vi "mediaBalls_v2.vi"(7 "cameras array":dbl[](array[numeric]), 9 "Field Size":T2, 10 "grSim?":bool=TRUE, 11 "Array Ball Pose + CamID":T1(array[cluster])) -> (2 "No cameras?":bool, 3 "Ball out":cluster{"x":dbl, "y":dbl})   [LabVIEW 2018]
panel:
  out "Array":i32[](array[numeric])
  in  "Cam Intersection Widht":u32=6
  in  "Cam Intersection Lenght":u32=6
  in  "cluster":cluster{"x":dbl, "y":dbl}
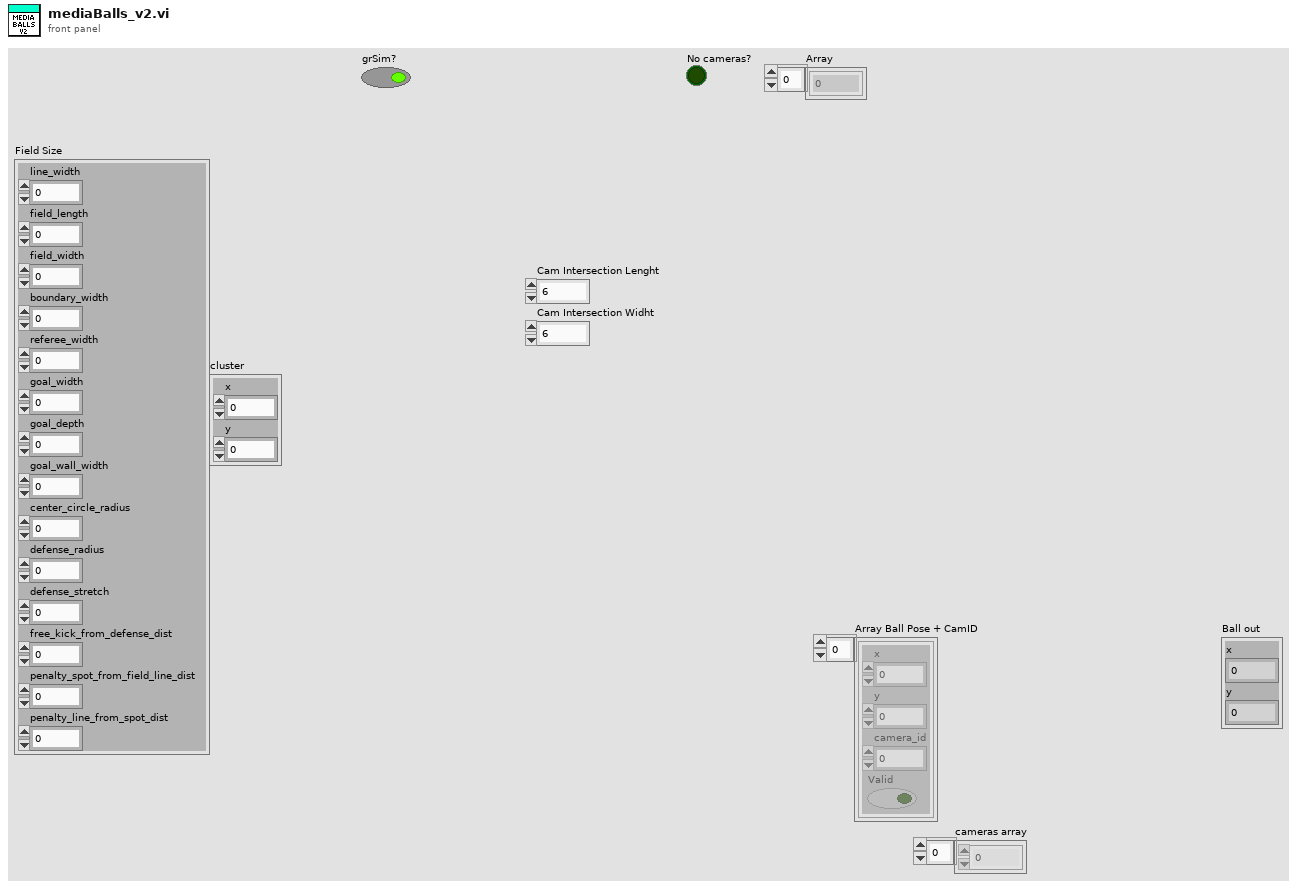
[diagram p1: front panel]
types:
  T1 = cluster{"x":sgl, "y":sgl, "camera_id":u32, "Valid":bool}[]
  T2 = cluster{"line_width":u32, "field_length":u32, "field_width":u32, "boundary_width":u32, "referee_width":u32, "goal_width":u32, "goal_depth":u32, "goal_wall_width":u32, "center_circle_radius":u32, "defense_radius":u32, "defense_stretch":u32, "free_kick_from_defense_dist":u32, "penalty_spot_from_field_line_dist":u32, "penalty_line_from_spot_dist":u32}
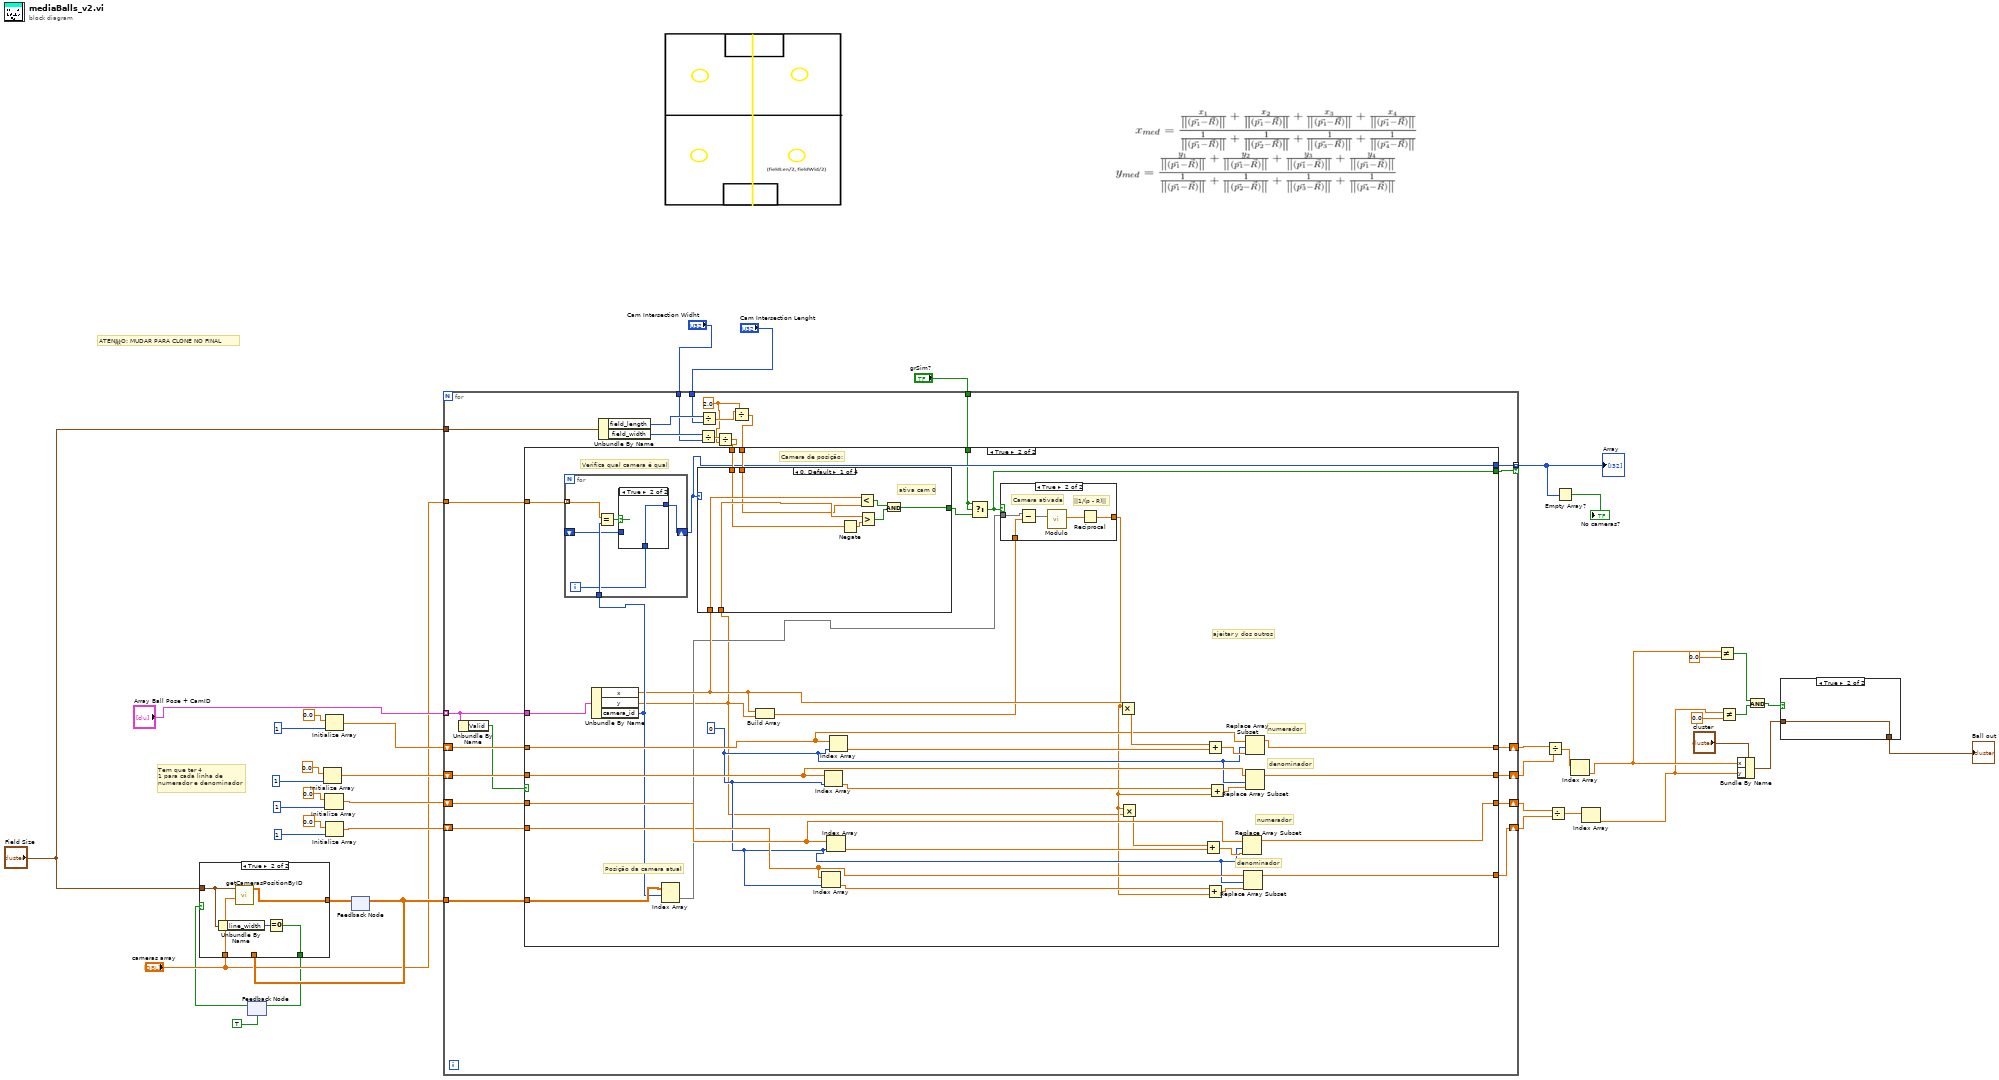
[diagram p0: block diagram]
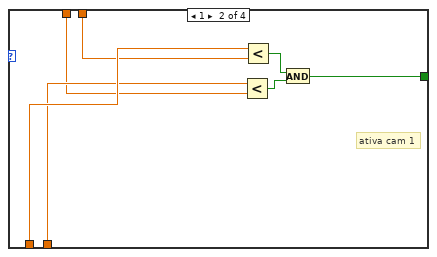
[diagram p5: hidden frame]
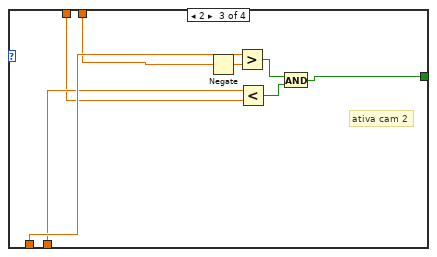
[diagram p6: hidden frame]
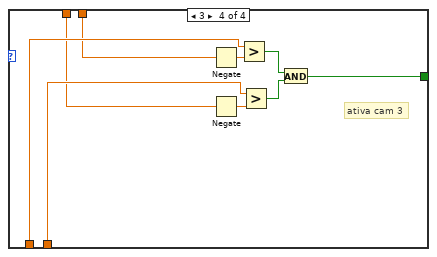
[diagram p7: hidden frame]
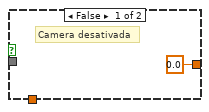
[diagram p9: hidden frame]
diagram:
  # "Tem que ter 4\n1 para cada linha de\nnumerador e denominador"
  # "ATEN敲O: MUDAR PARA CLONE NO FINAL"
  n1 = feedback #1(TRUE) -> (w2:bool)
  n2 = Initialize Array(0.0 ("element"), 1 ("dimension size")) -> (w32:dbl[])
  n3 = Initialize Array(0.0 ("element"), 1 ("dimension size")) -> (w31:dbl[])
  n4 = Initialize Array(0.0 ("element"), 1 ("dimension size")) -> (w33:dbl[])
  n5 = Initialize Array(0.0 ("element"), 1 ("dimension size")) -> (w30:dbl[])
  n6 = feedback #2() -> (w11:dbl[][])  [unwired: 1 in]
  n7 = case shown="True" w2 {
    selector: w2 -> [w42 _]
    tunnel: "Field Size" -> [_ w46]
    tunnel: [w43 w48] -> w12
    tunnel: w11 -> [w43 _]
    tunnel: "cameras array" -> [_ w47]
    tunnel: [w42 w44] -> w1
    frame False {
    }
    frame True {
      n8 = Unbundle By Name(w46) -> ("line_width"=w45:u32)
      n9 = call "getCamerasPositionByID.vi"("cameras id"=w47, "Field Size 2"=w46) -> ("Cameras Positions"=w48:dbl[][])  [unwired: 9 in]
      n10 = Equal To 0?(x=w45) -> (x = 0?=w44:bool)
    }
  }
  n11 = feedback-in #1(w1) -> ()
  n12 = feedback-in #2(w12) -> ()
  n13 = for {
    tunnel: "Array Ball Pose + CamID" -> [w50] mode=indexing
    tunnel: w11 -> [w73]
    shift-right: [w72] -> w29
    shift-left: w33 -> [w66]
    shift-right: [w71] -> w28
    shift-left: w32 -> [w65]
    shift-right: [w70] -> w27
    shift-left: w31 -> [w68]
    shift-right: [w69] -> w26
    shift-left: w30 -> [w67]
    tunnel: "cameras array" -> [w64]
    tunnel: "Cam Intersection Widht" -> [w61]
    tunnel: "Cam Intersection Lenght" -> [w60]
    tunnel: "Field Size" -> [w59]
    tunnel: "grSim?" -> [w58]
    tunnel: [w57] -> w7 mode=indexing if=w56
    w51 = 2.0
    n14 = Unbundle By Name(w50) -> ("Valid"=w49:bool)
    n15 = Unbundle By Name(w59) -> ("field_length"=w63:u32, "field_width"=w62:u32)
    n16 = Divide(x=w62, y=w61) -> (x/y=w53:dbl)
    n17 = Divide(x=w63, y=w60) -> (x/y=w55:dbl)
    n18 = Divide(x=w53, y=w51) -> (x/y=w52:dbl)
    n19 = Divide(x=w55, y=w51) -> (x/y=w54:dbl)
    n20 = case shown="True" w49 {
      tunnel: w73 -> [_ w111]
      tunnel: [w77 w101] -> w72
      tunnel: [w76 w100] -> w71
      tunnel: [w75 w99] -> w70
      tunnel: [w74 w98] -> w69
      tunnel: w68 -> [w75 w97]
      tunnel: w67 -> [w74 w96]
      tunnel: w66 -> [w77 w95]
      tunnel: w65 -> [w76 w94]
      tunnel: w50 -> [_ w91]
      tunnel: w64 -> [_ w89]
      tunnel: w52 -> [_ w88]
      tunnel: w54 -> [_ w87]
      tunnel: w58 -> [_ w80]
      tunnel: [_ w81] -> w57
      tunnel: [_ w78] -> w56
      frame False {
      }
      frame True {
        w93 = 0 ("index")
        # "Verifica qual camera é qual"
        # "Camera de posição:"
        # "ajeitar y dos outros"
        # "denominador"
        # "numerador"
        # "denominador"
        # "numerador"
        # "Posição da camera atual"
        n21 = Unbundle By Name(w91) -> ("x"=w86:sgl, "y"=w82:sgl, "camera_id"=w90:u32)
        n22 = for {
          tunnel: w90 -> [w149]
          shift-right: [w146] -> w81
          shift-left: _ -> [w145]
          tunnel: w89 -> [w144] mode=indexing
          i -> [w147]
          n23 = Equal?(x=w144, y=w149) -> (x = y?=w148:bool)
          n24 = case shown="True" w148 {
            tunnel: w147 -> [_ w151]
            tunnel: [w150 w151] -> w146
            tunnel: w145 -> [w150 _]
            frame False {
            }
            frame True {
            }
          }
        }
        n25 = Index Array(array=w111, index (row)=w90) -> (element=w85:dbl[])  [unwired: 1 in]
        n26 = case shown="0, Default" w81 {
          tunnel: w86 -> [w116 w124 w131 w139]
          tunnel: w82 -> [w115 w123 w130 w138]
          tunnel: [w112 w120 w127 w135] -> w79
          tunnel: w87 -> [w114 w122 w129 w137]
          tunnel: w88 -> [w113 w121 w128 w136]
          frame 0, Default {
            # "ativa cam 0"
            n27 = Negate(x=w113) -> (-x=w117:dbl)
            n28 = Less?(x=w116, y=w114) -> (x < y?=w119:bool)
            n29 = Greater?(x=w115, y=w117) -> (0:w118:bool)
            n30 = And(x=w119, y=w118) -> (x .and. y?=w112:bool)
          }
          frame 1 {
            # "ativa cam 1"
            n31 = Less?(x=w123, y=w121) -> (x < y?=w126:bool)
            n32 = Less?(x=w124, y=w122) -> (x < y?=w125:bool)
            n33 = And(x=w125, y=w126) -> (x .and. y?=w120:bool)
          }
          frame 2 {
            # "ativa cam 2"
            n34 = Negate(x=w129) -> (-x=w134:dbl)
            n35 = Greater?(x=w131, y=w134) -> (0:w133:bool)
            n36 = Less?(x=w130, y=w128) -> (x < y?=w132:bool)
            n37 = And(x=w133, y=w132) -> (x .and. y?=w127:bool)
          }
          frame 3 {
            # "ativa cam 3"
            n38 = Negate(x=w137) -> (-x=w143:dbl)
            n39 = Negate(x=w136) -> (-x=w142:dbl)
            n40 = Greater?(x=w139, y=w143) -> (0:w140:bool)
            n41 = Greater?(x=w138, y=w142) -> (0:w141:bool)
            n42 = And(x=w140, y=w141) -> (x .and. y?=w135:bool)
          }
        }
        n43 = Build Array(w86, w82) -> (w84:sgl[])
        n44 = Index Array(array=w96, index=w93) -> (element=w102:dbl)
        n45 = Index Array(array=w94, index=w93) -> (element=w104:dbl)
        n46 = Index Array(array=w97, index=w93) -> (element=w103:dbl)
        n47 = Index Array(array=w95, index=w93) -> (element=w105:dbl)
        n48 = Select(t=w80, s=w80, f=w79) -> (s? t:f=w78:bool)
        n49 = case shown="True" w78 {
          tunnel: [0.0 w156] -> w83
          tunnel: w85 -> [_ w155]
          tunnel: w84 -> [_ w154]
          frame False {
            # "Camera desativada"
          }
          frame True {
            # "Camera ativada"
            # "||1/(p - R)||"
            n50 = Subtract(x=w155, y=w154) -> (x-y=w153:dbl[])
            n51 = call "Modulo.vi"("2D vector"=w153) -> ("Modulo"=w157:dbl)  [unwired: 10 in]
            n52 = Reciprocal(x=w157) -> (1/x=w156:dbl)
          }
        }
        n53 = Multiply(x=w83, y=w86) -> (x*y=w110:dbl)
        n54 = Multiply(x=w83, y=w82) -> (x*y=w92:dbl)
        n55 = Add(x=w92, y=w103) -> (x+y=w107:dbl)
        n56 = Add(x=w102, y=w83) -> (x+y=w106:dbl)
        n57 = Add(x=w110, y=w105) -> (x+y=w109:dbl)
        n58 = Add(x=w104, y=w83) -> (x+y=w108:dbl)
        n59 = Replace Array Subset(array=w97, new element=w107, index=w93) -> (w99:dbl[])
        n60 = Replace Array Subset(array=w96, new element=w106, index=w93) -> (w98:dbl[])
        n61 = Replace Array Subset(array=w95, new element=w109, index=w93) -> (w101:dbl[])
        n62 = Replace Array Subset(array=w94, new element=w108, index=w93) -> (w100:dbl[])
      }
    }
  }
  "Array" <- w7
  n63 = Divide(x=w29, y=w28) -> (x/y=w18:dbl[])
  n64 = Divide(x=w27, y=w26) -> (x/y=w16:dbl[])
  n65 = Empty Array?(array=w7) -> (empty?=→"No cameras?":bool)
  n66 = Index Array(array=w18) -> (element=w17:dbl)  [unwired: 1 in]
  n67 = Index Array(array=w16) -> (element=w15:dbl)  [unwired: 1 in]
  n68 = Not Equal?(x=w17, y=0.0) -> (x != y?=w23:bool)
  n69 = Not Equal?(x=w15, y=0.0) -> (x != y?=w22:bool)
  n70 = Bundle By Name(cluster="cluster", "x"=w17, "y"=w15) -> (w20:cluster{"x":dbl, "y":dbl})
  n71 = And(x=w23, y=w22) -> (x .and. y?=w21:bool)
  n72 = case shown="True" w21 {
    tunnel: [w158 w159] -> w14
    tunnel: w20 -> [w158 w159]
    frame False {
    }
    frame True {
    }
  }
  "Ball out" <- w14
